vi "dataInitilize.vi"(8 "error in (no error)":errorcluster, 11 "LaguerreDeconClass in":refnum<class "LaguerreDeconEngineClass.lvclass">) -> (0 "error out":errorcluster, 3 "LaguerreDeconClass out":refnum<class "LaguerreDeconEngineClass.lvclass">)   [LabVIEW 2020, in "LaguerreDeconEngineClass.lvclass"]
uses:
  LaguerreDeconEngineClass.lvclass
  LaguerreDeconEngineClass.lvclass/LaguerreDeconEngineClass.ctl
  LaguerreDeconLib.lvlib
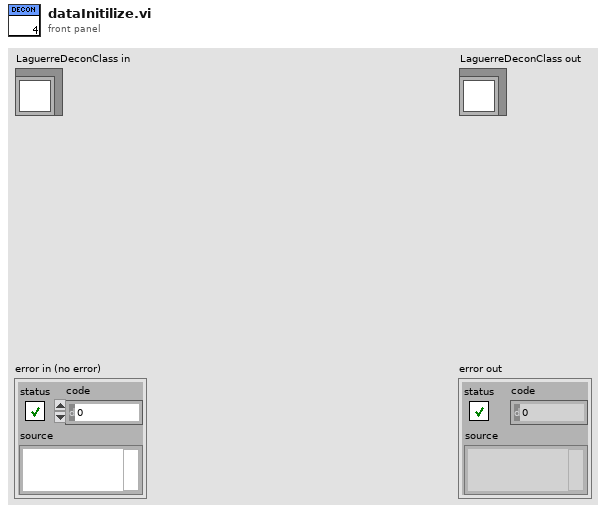
[diagram p1: front panel]
types:
  T1 = cluster{"LGBasisRows":u32, "LGBasisCols":u32, "vvRows":u32, "vvCols":u32, "DRows":u32, "DCols":u32, "LHS_Multi_Rows":u32, "LHS_Multi_Cols":u32, "RHS_Multi_Rows":u32, "RHS_Multi_Cols":u32, "lam length":u32, "LCs length":u32}
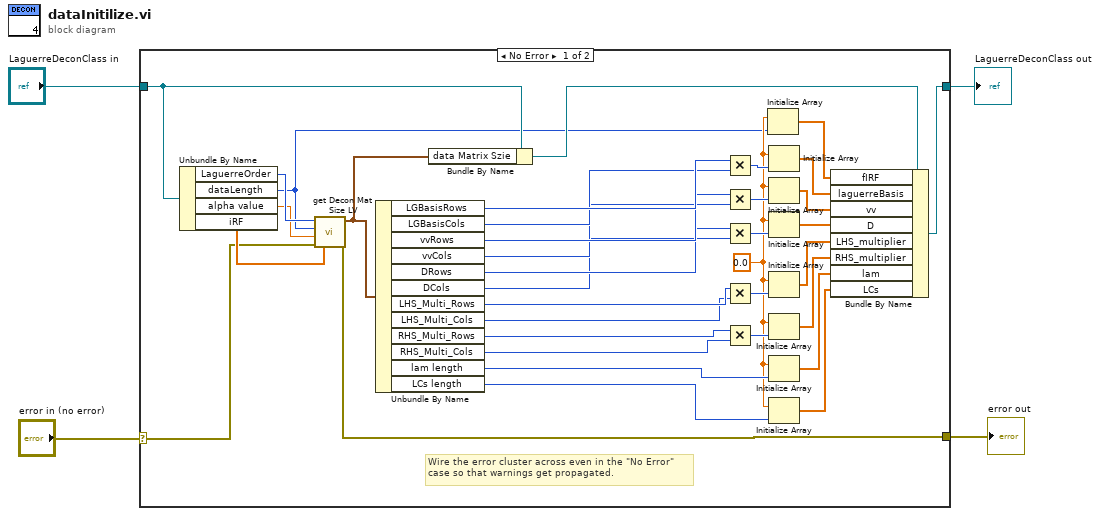
[diagram p0: block diagram]
diagram:
  n1 = case shown="No Error" "error in (no error)" {
    selector: "error in (no error)" -> [w14 w42]
    tunnel: [w13 w42] -> w3
    tunnel: [w24 w41] -> w1
    tunnel: "LaguerreDeconClass in" -> [w8 w41]
    frame No Error {
      w7 = 0.0 ("element")
      # "Wire the error cluster across even in the \"No Error\"\ncase so that warnings get propagated."
      n2 = Unbundle By Name(w8) -> ("LaguerreOrder"=w40:u32, "dataLength"=w6:u32, "alpha value"=w39:dbl, "iRF"=w38:dbl[])
      n3 = call "get Decon Mat Size LV.vi"("iRF_array"=w38, "error in (no error)"=w14, "alpha"=w39, "dataLength"=w6, "laguerreOrder"=w40) -> ("error out"=w13:errorcluster, "daat Matrix Szie"=w10:T1)  [unwired: 5 in]
      n4 = Unbundle By Name(w10) -> ("LGBasisRows"=w37:u32, "LGBasisCols"=w36:u32, "vvRows"=w35:u32, "vvCols"=w34:u32, "DRows"=w33:u32, "DCols"=w32:u32, "LHS_Multi_Rows"=w31:u32, "LHS_Multi_Cols"=w17:u32, "RHS_Multi_Rows"=w16:u32, "RHS_Multi_Cols"=w30:u32, "lam length"=w12:u32, "LCs length"=w11:u32)
      n5 = Bundle By Name(cluster=w8, "data Matrix Szie"=w10) -> (w9:refnum<class "LaguerreDeconEngineClass.lvclass">)
      n6 = Multiply(x=w37, y=w36) -> (x*y=w29:u32)
      n7 = Multiply(x=w35, y=w34) -> (x*y=w28:u32)
      n8 = Multiply(x=w33, y=w32) -> (x*y=w27:u32)
      n9 = Multiply(x=w31, y=w17) -> (x*y=w26:u32)
      n10 = Multiply(x=w16, y=w30) -> (x*y=w25:u32)
      n11 = Initialize Array(w7, w6) -> (w5:dbl[])
      n12 = Initialize Array(w7, w29) -> (w22:dbl[])
      n13 = Initialize Array(w7, w28) -> (w20:dbl[])
      n14 = Initialize Array(w7, w27) -> (w21:dbl[])
      n15 = Initialize Array(w7, w26) -> (w19:dbl[])
      n16 = Initialize Array(w7, w25) -> (w18:dbl[])
      n17 = Initialize Array(w7, w12) -> (w23:dbl[])
      n18 = Initialize Array(w7, w11) -> (w15:dbl[])
      n19 = Bundle By Name(cluster=w9, "fIRF"=w5, "laguerreBasis"=w22, "vv"=w20, "D"=w21, "LHS_multiplier"=w19, "RHS_multiplier"=w18, "lam"=w23, "LCs"=w15) -> (w24:refnum<class "LaguerreDeconEngineClass.lvclass">)
    }
    frame Error {
    }
  }
  "error out" <- w3
  "LaguerreDeconClass out" <- w1
